vi "ProdaNG.ProductComponent.Get.vi"(8 "error in (no error)":errorcluster, 9 "serialNumber":string, 10 "wabcoNumber":string, 11 "dbHandle":i32) -> (0 "error out":errorcluster, 2 "ProdComponents":T1[](array[typedef]), 3 "dbHandle out":i32)   [LabVIEW 2016]
doc: "This function returns a product structure for a product, which is identified by a part and a serial number.\nImportant information: The field 'individual' was taken over from the field 'allgemein' of the legacy data directly. Because of this most products have the value 0 further on and only a few the value 1. \nParameter:\nhandle is an Integer, which is returned by the function Login() at the creation of a new connection.\nwabcoPartId is the Id of the part.\nserialNumber is the serial number of the product for the part above.\nproduct is a pointer on a product structure, which is filled if the returncode is 0. The structure must be defined in the calling program.\n\nReturncodes:\n0 No error\n< 0 ORACLE Error code\n6 (ERROR_INVALID_HANDLE) in case of an invalid handle\n1403 Record does not exist"
uses:
  Controls/ProdaNG.ProductComponent.ctl
  Controls/ProdaNG.ProductionLineSize.ctl
  <vilib>/Utility/importsl/GetValueByPointer/datatype.ctl
  <vilib>/Utility/importsl/GetValueByPointer/GetValueByPointer.xnode
  prodllNG.dll
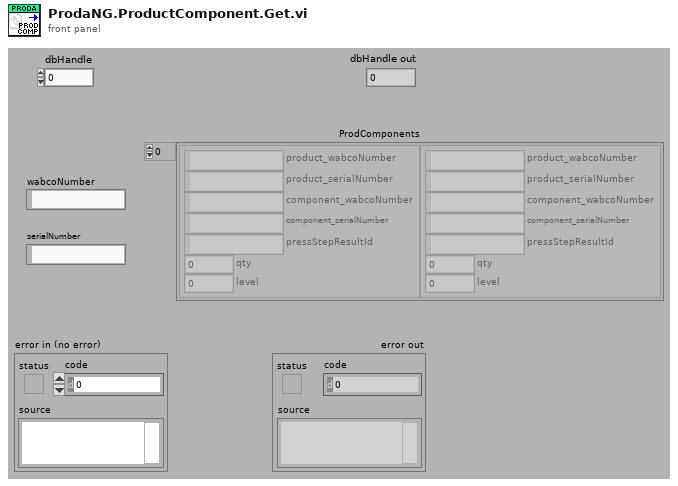
[diagram p1: front panel]
types:
  T1 = typedef "ProdaNG.ProductComponent.ctl" = cluster{"product_wabcoNumber":string, "product_serialNumber":string, "component_wabcoNumber":string, "component_serialNumber":string, "pressStepResultId":string, "qty":i32, "level":i32}
  T2 = typedef "ProdaNG.ProductionLineSize.ctl" = cluster{"product_wabcoNumber":i32, "product_serialNumber":i32, "component_wabcoNumber":i32, "component_serialNumber":i32, "pressStepResultId":i32, "qty":i32, "level":i32}
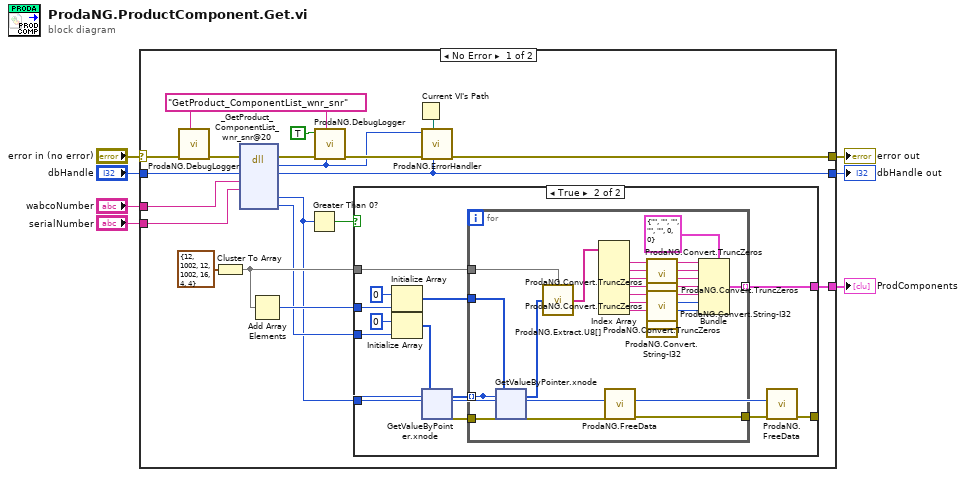
[diagram p0: block diagram]
diagram:
  n1 = case shown="No Error" "error in (no error)" {
    selector: "error in (no error)" -> [w25 w96]
    tunnel: [w26 w96] -> w6
    tunnel: "dbHandle" -> [w19 w95]
    tunnel: [w20 w95] -> w4
    tunnel: "wabcoNumber" -> [w21 _]
    tunnel: "serialNumber" -> [w22 _]
    tunnel: [w11 _] -> w1
    frame No Error {
      w15 = "GetProduct_ComponentList_wnr_snr" ("cmd")
      n2 = call "ProdaNG.DebugLogger.vi"("cmd"=w15, "error in (no error)"=w25) -> ("error out"=w18:errorcluster)  [unwired: 9 in]
      n3 = Cluster To Array(cluster=T2 {"product_wabcoNumber"=12, "product_serialNumber"=1002, "component_wabcoNumber"=12, "component_serialNumber"=1002, "pressStepResultId"=16, "qty"=4, "level"=4} ("ProductComponentSize")) -> (array=w13:i32[])
      n4 = dll-call lib="D:/Maszup/WABCO/SVN/BSV/SOFTWARE-LASER/sources/Database/ProdaNG/prodllNG.dll" fn="_GetProduct_ComponentList_wnr_snr@20" ("ProDll wrapper.dll:wrapper_GetWabcoParts_init")(error in=w18, "dbHandle"=w19, "wabcoNumber"=w21, "serialNumber"=w22) -> (error out=w17:errorcluster, "return type"=w23:i32, "dbHandle"=w20:i32, "product_component_wnr_snr"=w9:i32, "countPtr"=w10:u32)  [unwired: 6 in, 1 out]
      n5 = Add Array Elements(numeric array=w13) -> (sum=w14:i32)
      n6 = Greater Than 0?(x=w9) -> (x > 0?=w8:bool)
      n7 = call "ProdaNG.DebugLogger.vi"("return type"=w23, "cmd"=w15, "error in (no error)"=w17, "done? (F)"=TRUE) -> ("error out"=w24:errorcluster)  [unwired: 7 in]
      n8 = case shown="True" w8 {
        tunnel: w14 -> [_ w34]
        tunnel: w13 -> [_ w33]
        tunnel: w9 -> [_ w31]
        tunnel: [_ w30] -> w11
        tunnel: [_ w29] -> _
        tunnel: w10 -> [_ w28]
        frame False {
        }
        frame True {
          n9 = Initialize Array(u8 0 ("element"), w34) -> (w35:u8[])
          n10 = Initialize Array(u32 0 ("element"), w28) -> (w40:u32[])
          n11 = xnode "GetValueByPointer.xnode"("Pointer"=w31, "InputType"=w40) -> ("Output"=w37:u32[], "ErrorOut"=w38:errorcluster)  [unwired: 2 in]
          n12 = for {
            tunnel: w38 -> [w64]
            tunnel: w37 -> [w44] mode=indexing
            tunnel: w35 -> [w63]
            tunnel: w33 -> [w47]
            tunnel: [w46] -> w30 mode=indexing
            tunnel: [w43] -> w32
            n13 = xnode "GetValueByPointer.xnode"("Pointer"=w44, "InputType"=w63, "ErrorIn"=w64) -> ("Output"=w49:u8[], "ErrorOut"=w45:errorcluster)  [unwired: 1 in]
            n14 = call "ProdaNG.Extract.U8[].vi"("unsigned byte array"=w49, "Sizes"=w47) -> ("Elements"=w48:string[])
            n15 = Index Array(array=w48) -> (element #1=w51:string, element #2=w50:string, element #3=w61:string, element #4=w58:string, element #5=w55:string, element #6=w57:string, element #7=w41:string)  [unwired: 7 in]
            n16 = call "ProdaNG.FreeData.vi"("error in (no error)"=w45, "Pointers"=w44) -> ("error out"=w43:errorcluster)  [unwired: 9 in]
            n17 = call "ProdaNG.Convert.TruncZeros.vi"("string with \\0s"=w51) -> ("LV string"=w53:string)  [unwired: 10 in]
            n18 = call "ProdaNG.Convert.TruncZeros.vi"("string with \\0s"=w50) -> ("LV string"=w52:string)  [unwired: 10 in]
            n19 = call "ProdaNG.Convert.TruncZeros.vi"("string with \\0s"=w61) -> ("LV string"=w60:string)  [unwired: 10 in]
            n20 = call "ProdaNG.Convert.TruncZeros.vi"("string with \\0s"=w58) -> ("LV string"=w59:string)  [unwired: 10 in]
            n21 = call "ProdaNG.Convert.TruncZeros.vi"("string with \\0s"=w55) -> ("LV string"=w54:string)  [unwired: 10 in]
            n22 = call "ProdaNG.Convert.String-I32.vi"("unsigned byte string"=w57) -> ("32bit integer"=w56:i32)  [unwired: 10 in]
            n23 = call "ProdaNG.Convert.String-I32.vi"("unsigned byte string"=w41) -> ("32bit integer"=w42:i32)  [unwired: 10 in]
            n24 = Bundle(cluster=T1 {"product_wabcoNumber"="", "product_serialNumber"="", "component_wabcoNumber"="", "component_serialNumber"="", "pressStepResultId"="", "qty"=0, "level"=0} ("Product_Component_wnr_str"), "product_wabcoNumber"=w53, "product_serialNumber"=w52, "component_wabcoNumber"=w60, "component_serialNumber"=w59, "pressStepResultId"=w54, "qty"=w56, "level"=w42) -> (w46:T1)
          }
          n25 = call "ProdaNG.FreeData.vi"("error in (no error)"=w32, "Pointers"=w31) -> ("error out"=w29:errorcluster)  [unwired: 9 in]
        }
      }
      n26 = Current VI's Path() -> (path=w27:path)
      n27 = call "ProdaNG.ErrorHandler.vi"("dbHandleIn"=w20, "Path"=w27, "error in"=w24, "output_parameter"=w23) -> ("error out"=w26:errorcluster)  [unwired: 7 in]
    }
    frame Error {
    }
  }
  "error out" <- w6
  "dbHandle out" <- w4
  "ProdComponents" <- w1
